vi "不同坐标轴.vi"() -> ()   [LabVIEW 2022 SP3]
doc: "本VI是为《我和LabVIEW》一书编写的示例。\n关于本书的介绍请参考网页：\nhttp://ruanqizhen.spaces.live.com/blog/cns!5852D4F797C53FB6!4310.entry"
panel:
  out "波形":dbl[][](graph) caption="(Y) Multi Plot 2"
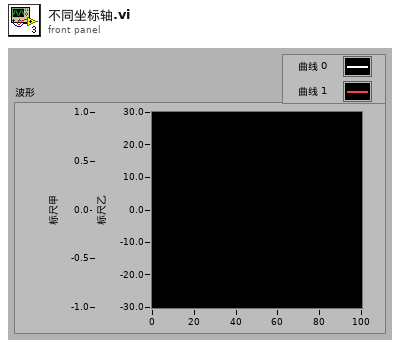
[diagram p1: front panel]
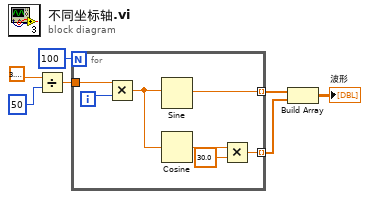
[diagram p0: block diagram]
diagram:
  n1 = Divide(x=3.141592653589793, y=50) -> (x/y=w5:dbl)
  n2 = for {
    N: 100 -> [_]
    tunnel: w5 -> [w14]
    tunnel: [w11] -> w3 mode=indexing
    tunnel: [w8] -> w2 mode=indexing
    i -> [w13]
    n3 = Multiply(x=w14, y=w13) -> (x*y=w12:dbl)
    n4 = Sine(x=w12) -> (sin(x)=w11:dbl)
    n5 = Cosine(x=w12) -> (cos(x)=w10:dbl)
    n6 = Multiply(x=w10, y=30.0) -> (x*y=w8:dbl)
  }
  n7 = Build Array(w3, w2) -> (→"波形":dbl[][])
